vi "Read TCP Configs.vi"(8 "error in (no error)":errorcluster, 10 "Item Ref in":T2 format="%.0x", 11 "Refnum in":T1) -> (0 "error out":errorcluster, 2 "Item Ref out":T2 format="%.0x", 3 "Refnum out":T1)   [LabVIEW 2015, in "Modbus Master System Explorer.lvlib"]
uses:
  Modbus Master System Explorer.lvlib
  <vilib>/NI Veristand/Custom Device API/Custom Device Item Ref.ctl
  <vilib>/Utility/config.llb/Config Data RefNum.ctl
  <vilib>/Utility/config.llb/Read Key (String).vi
  <vilib>/Utility/config.llb/Read Key (U32).vi
  <vilib>/Utility/config.llb/Read Key (I32).vi
  <vilib>/Utility/config.llb/NI_LVConfig.lvlib
  <vilib>/NI VeriStand/Custom Device API/Custom Device API.lvlib
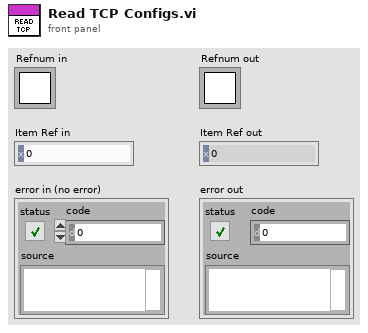
[diagram p1: front panel]
types:
  T1 = typedef "NI_LVConfig.lvlib/Config Data RefNum.ctl" = refnum<k1>
  T2 = typedef "Custom Device API.lvlib/Custom Device Item Ref.ctl" = u64
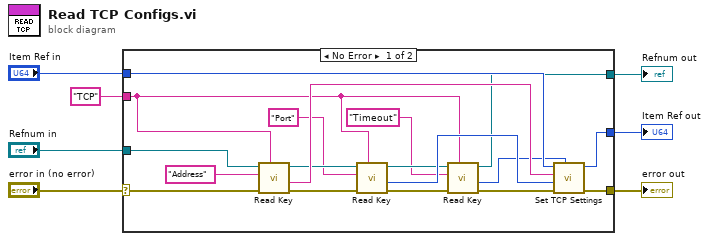
[diagram p0: block diagram]
diagram:
  n1 = case shown="No Error" "error in (no error)" {
    selector: "error in (no error)" -> [w23 w26]
    tunnel: [w25 w27] -> w7
    tunnel: [w24 w26] -> w6
    tunnel: "TCP" ("section") -> [w12 _]
    tunnel: [w10 w28] -> w3
    tunnel: "Item Ref in" -> [w16 w27]
    tunnel: "Refnum in" -> [w15 w28]
    frame No Error {
      n2 = call-poly <vilib>:"Read Key.vi"("section"=w12, "error in (no error)"=w23, "key"="Address", "refnum"=w15) -> ("error out"=w21:errorcluster, "value"=w20:string, "refnum out"=w19:T1)  [unwired: 4 in, 1 out]
      n3 = call-poly <vilib>:"Read Key.vi"("section"=w12, "error in (no error)"=w21, "key"="Port", "refnum"=w19) -> ("error out"=w14:errorcluster, "value"=w17:u32, "refnum out"=w11:T1)  [unwired: 4 in, 1 out]
      n4 = call-poly <vilib>:"Read Key.vi"("section"=w12, "error in (no error)"=w14, "key"="Timeout", "refnum"=w11) -> ("error out"=w13:errorcluster, "value"=w8:i32, "refnum out"=w10:T1)  [unwired: 4 in, 1 out]
      n5 = call "Set TCP Settings.vi"("Timeout"=w8, "error in (no error)"=w13, "Port"=w17, "Address"=w20, "Item Ref in"=w16) -> ("error out"=w24:errorcluster, "Item Ref out"=w25:T2)  [unwired: 5 in]
    }
    frame Error {
    }
  }
  "Item Ref out" <- w7
  "error out" <- w6
  "Refnum out" <- w3
